vi "signal_mapping_lock-in-measurement.vi"() -> ()   [LabVIEW 2024]
uses:
  <vilib>/Utility/file.llb/Write Delimited Spreadsheet (string).vi
  <vilib>/Utility/file.llb/Write Delimited Spreadsheet (DBL).vi
  <vilib>/Analysis/NI_AALBase.lvlib
panel:
  in  "Set Sensitivities":bool
  in  "A Sensitivity":u16(ring)=20 items=["1 nV/fA", "2 nV/fA", "5 nV/fA", "10 nV/fA", "20 nV/fA", "50 nV/fA", "100 nV/fA", "200 nV/fA", "500 nV/fA", "1 uV/pA", "2 uV/pA", "5 uV/pA", "10 uV/pA", "20 uV/pA", "50 uV/pA", "100 uV/pA", "200 uV/pA", "500 uV/pA", "1 mV/nA", "2 mV/nA", "5 mV/nA", "10 mV/nA", "20 mV/nA", "50 mV/nA", "100 mV/nA", "200 mV/nA", "500 mV/nA", "1 V/uA"]
  in  "B Sensitivity":u16(ring)=20 items=["1 nV/fA", "2 nV/fA", "5 nV/fA", "10 nV/fA", "20 nV/fA", "50 nV/fA", "100 nV/fA", "200 nV/fA", "500 nV/fA", "1 uV/pA", "2 uV/pA", "5 uV/pA", "10 uV/pA", "20 uV/pA", "50 uV/pA", "100 uV/pA", "200 uV/pA", "500 uV/pA", "1 mV/nA", "2 mV/nA", "5 mV/nA", "10 mV/nA", "20 mV/nA", "50 mV/nA", "100 mV/nA", "200 mV/nA", "500 mV/nA", "1 V/uA"]
  in  "Lock-In Num Avgs":i32
  out "错误输出":errorcluster
  out "AUX-ADC4 (V)":sgl format="%.3f"
  out "AUX-ADC3 (V)":sgl format="%.3f"
  out "AUX-ADC1 (V)":sgl format="%.3f"
  out "AUX-ADC2 (V)":sgl format="%.3f"
  in  "OE1022D 2":refnum<visa-resource-name> caption="OE1022D"
  out "序列号":string
  in  "ms to wait after move":u32=1
  in  "ANC300 address":refnum<visa-resource-name>="COM8"
  in  "Snake":bool
  in  "File to save to":path
  in  "Select Scan Type":u16(ring)=1 items=["line scan", "rectangular scan"]
  in  "scan points":i32
  in  "y end":i32
  in  "x end":i32
  in  "y start":i32
  in  "x start":i32
  in  "y scan points":i32
  in  "x scan points":i32
  in  "y scan size":i32
  in  "x scan size":i32
  in  "y center":i32
  in  "x center":i32
  # "Scaning Setup"
  # "Rectangular Scan Parameters"
  # "Line Scan Parameters"
  # "Measurement Setup"
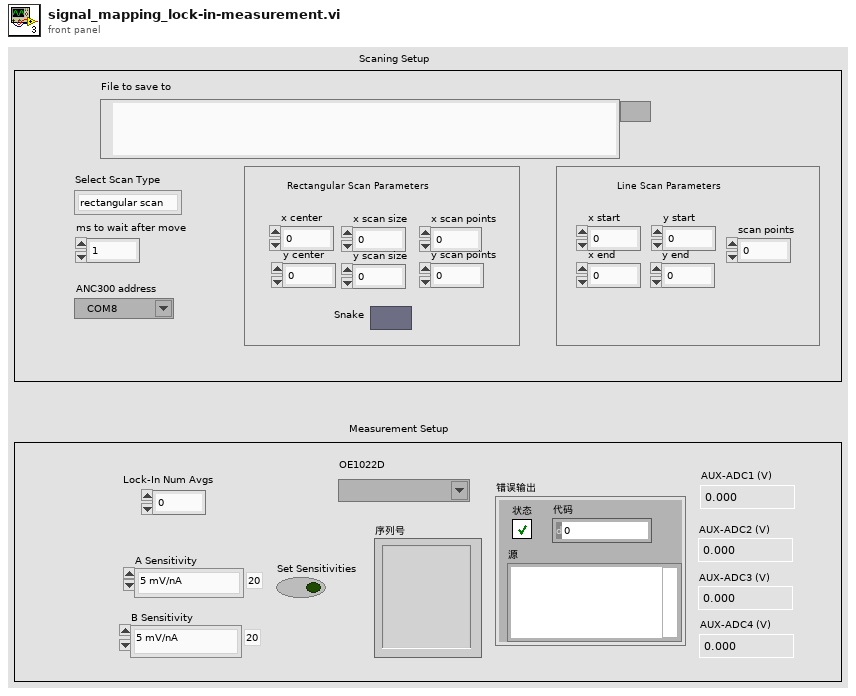
[diagram p1: front panel]
types:
  T1 = cluster{"error ":bool, "error number":i32, "error code":string}
  T2 = cluster{"AD1":dbl[], "AD2":dbl[], "AD3":dbl[], "AD4":dbl[]}
  T3 = cluster{"XB":dbl[], "YB":dbl[], "FrequencyB":dbl[], "NoiseB":dbl[], "Xh1B":dbl[], "Yh1B":dbl[], "Xh2B":dbl[], "Yh2B":dbl[], "Xh2B":dbl[]}
  T4 = cluster{"XA":dbl[], "YA":dbl[], "FrequencyA":dbl[], "NoiseA":dbl[], "Xh1A":dbl[], "Yh1A":dbl[], "Xh2A":dbl[], "Yh2A":dbl[]}
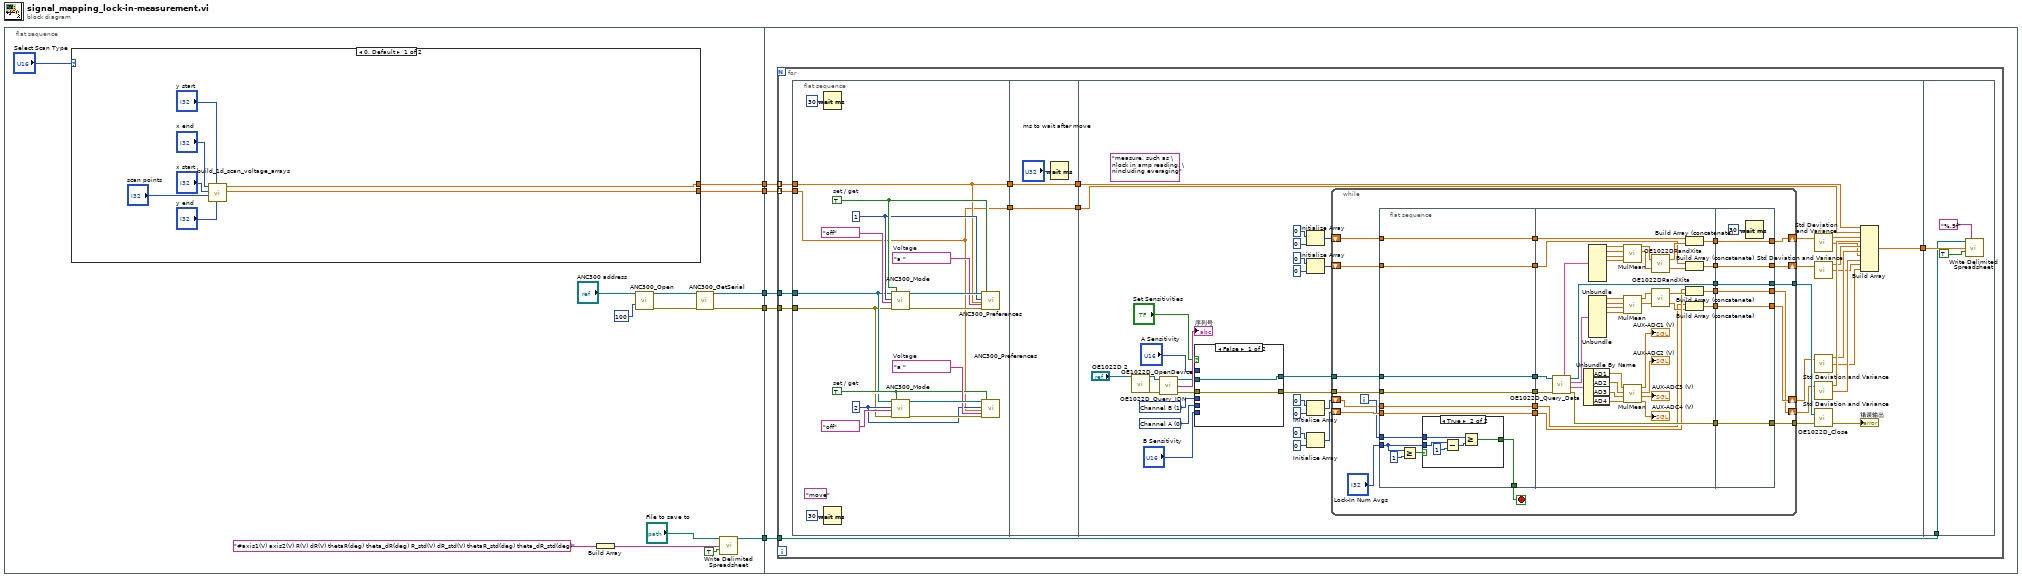
[diagram p0: block diagram]
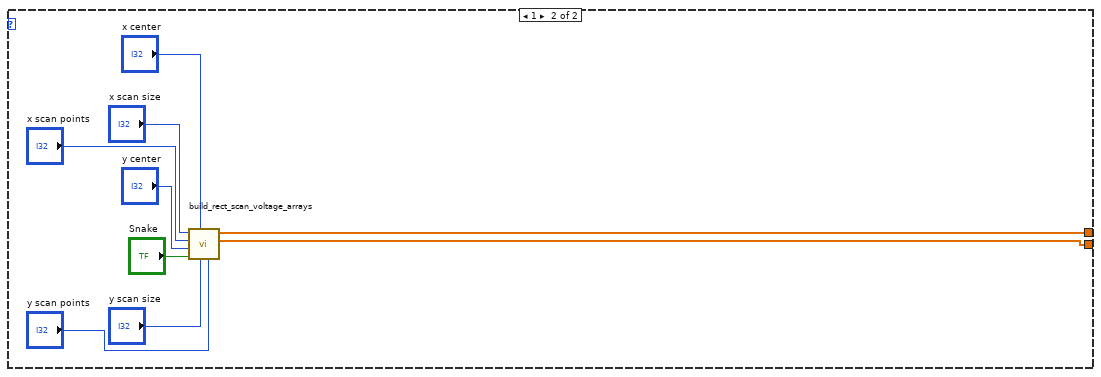
[diagram p2: hidden frame]
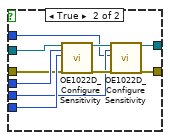
[diagram p3: hidden frame]
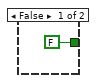
[diagram p4: hidden frame]
diagram:
  n1 = flat-sequence {
    tunnel: [w18] -> w5
    tunnel: [w19] -> w4
    tunnel: [w13] -> w3
    tunnel: [w12] -> w2
    tunnel: [w6] -> w1
    tunnel: w5 -> [w40]
    tunnel: w4 -> [w39]
    tunnel: w3 -> [w38]
    tunnel: w2 -> [w37]
    tunnel: w1 -> [w36]
    frame #0 {
      n2 = case shown="0, Default" "Select Scan Type" {
        tunnel: [w20 w35] -> w19
        tunnel: [w21 w34] -> w18
        frame 0, Default {
          n3 = call "build_1d_scan_voltage_arrays.vi"("y end"="y end", "y start"="y start", "scan points"="scan points", "x start"="x start", "x end"="x end") -> ("y voltage array"=w20:dbl[], "x voltage array"=w21:dbl[])  [unwired: 5 in]
        }
        frame 1 {
          n4 = call "build_rect_scan_voltage_arrays.vi"("y scan points"="y scan points", "y scan size"="y scan size", "x center"="x center", "Snake"="Snake", "y center"="y center", "x scan points"="x scan points", "x scan size"="x scan size") -> ("y voltage array"=w35:dbl[], "x voltage array"=w34:dbl[])  [unwired: 3 in]
        }
      }
      n5 = Build Array("#axis1(V) axis2(V) R(V) dR(V) thetaR(deg) theta_dR(deg) R_std(V) dR_std(V) thetaR_std(deg) theta_dR_std(deg)") -> (w8:string[])
      n6 = call "ANC300_Open.vi"("ANC300 Communication Port In"="ANC300 address", "milliseconds to wait"=u32 100 ("millisecond timer value")) -> ("ANC300 Communication Port Out"=w14:refnum<visa-resource-name>, "error out"=w11:T1)  [unwired: 13 in, 3 out]
      n7 = call "ANC300_GetSerial.vi"("ANC300 Communication Port In"=w14, "error in"=w11) -> ("ANC300 Communication Port Out"=w13:refnum<visa-resource-name>, "error out"=w12:T1)  [unwired: 10 in, 6 out]
      n8 = call-poly <vilib>:"Write Delimited Spreadsheet.vi"("file path (dialog if empty)"="File to save to", "1D data"=w8, "append to file? (new file:F)"=TRUE) -> ("new file path (Not A Path if cancelled)"=w6:path)  [unwired: 11 in, 1 out]
    }
    frame #1 {
      n9 = for {
        tunnel: w40 -> [w50] mode=indexing
        tunnel: w39 -> [w49] mode=indexing
        tunnel: w38 -> [w48]
        tunnel: w37 -> [w47]
        tunnel: w36 -> [w41]
        n10 = flat-sequence {
          tunnel: w50 -> [w52]
          tunnel: w49 -> [w51]
          tunnel: w48 -> [w55]
          tunnel: w47 -> [w54]
          tunnel: [w52] -> w44
          tunnel: [w51] -> w43
          tunnel: [w70] -> w45
          tunnel: w44 -> [w70]
          tunnel: w43 -> [w69]
          tunnel: [w69] -> w42
          tunnel: [w108] -> w46
          tunnel: w45 -> [w100]
          tunnel: w42 -> [w99]
          tunnel: w46 -> [w219]
          tunnel: w41 -> [w217]
          frame #0 {
            w56 = 2
            w57 = 1
            w58 = TRUE  # set / get
            w60 = "a "  # Voltage
            w63 = TRUE  # set / get
            w66 = "a "  # Voltage
            (unwired) "move"
            n11 = Wait (ms)(milliseconds to wait=u32 30 ("2: ms to wait")) -> ()  [unwired: 1 out]
            n12 = Wait (ms)(milliseconds to wait=u32 30 ("1: ms to wait")) -> ()  [unwired: 1 out]
            n13 = call "ANC300_Mode.vi"("ANC300 Communication Port In"=w55, "Axis"=w57, "axis mode in"="off", "error in"=w54, "set / get"=w63) -> ("ANC300 Communication Port Out"=w68:refnum<visa-resource-name>, "error out"=w67:T1)  [unwired: 8 in, 5 out]
            n14 = call "ANC300_Mode.vi"("ANC300 Communication Port In"=w55, "Axis"=w56, "axis mode in"="off", "error in"=w54, "set / get"=w58) -> ("ANC300 Communication Port Out"=w62:refnum<visa-resource-name>, "error out"=w61:T1)  [unwired: 8 in, 5 out]
            n15 = call "ANC300_Preferences.vi"("ANC300 Communication Port In"=w68, "Axis"=w57, "value in"=w52, "parameter"=w66, "error in"=w67, "set / get"=w63) -> ()  [unwired: 6 in, 8 out]
            n16 = call "ANC300_Preferences.vi"("ANC300 Communication Port In"=w62, "Axis"=w56, "value in"=w51, "parameter"=w60, "error in"=w61, "set / get"=w58) -> ()  [unwired: 6 in, 8 out]
          }
          frame #1 {
            n17 = Wait (ms)(milliseconds to wait="ms to wait after move") -> ()  [unwired: 1 out]
          }
          frame #2 {
            w86 = u8 0 items=["Channel A", "Channel B"] ("OE1022D A/B")
            w92 = u8 1 items=["Channel A", "Channel B"] ("OE1022D A/B")
            (unwired) "measure, such as \nlock in amp reading, \nincluding everaging"
            n18 = call "OE1022D_OpenDevice.vi"("VISA resource name"="OE1022D 2") -> ("VISA资源名称输出"=w105:refnum<visa-resource-name>, "错误输出"=w106:errorcluster)  [unwired: 17 in]
            n19 = call "OE1022D_Query_IDN.vi"("错误输入（无错误）"=w106, "VISA resource name"=w105) -> ("错误输出"=w90:errorcluster, "序列号"=→"序列号":string, "VISA resource name out"=w89:refnum<visa-resource-name>)  [unwired: 1 in]
            n20 = case shown="False" "Set Sensitivities" {
              tunnel: w92 -> [_ w126]
              tunnel: "B Sensitivity" -> [_ w125]
              tunnel: w90 -> [w115 w124]
              tunnel: w89 -> [w116 w123]
              tunnel: [w116 w120] -> w88
              tunnel: [w115 w119] -> w87
              tunnel: w86 -> [_ w118]
              tunnel: "A Sensitivity" -> [_ w117]
              frame False {
              }
              frame True {
                n21 = call "OE1022D_Configure Sensitivity.vi"("VISA resource name"=w123, "OE1022D A/B"=w126, "Sensitivity"=w125, "error in (no error)"=w124) -> ("VISA resource name out"=w121:refnum<visa-resource-name>, "error out"=w122:errorcluster)  [unwired: 14 in]
                n22 = call "OE1022D_Configure Sensitivity.vi"("VISA resource name"=w121, "OE1022D A/B"=w118, "Sensitivity"=w117, "error in (no error)"=w122) -> ("VISA resource name out"=w120:refnum<visa-resource-name>, "error out"=w119:errorcluster)  [unwired: 14 in]
              }
            }
            n23 = Initialize Array(0, 0) -> (w114:i32[])
            n24 = Initialize Array(0, 0) -> (w94:i32[])
            n25 = Initialize Array(0, 0) -> (w93:i32[])
            n26 = Initialize Array(0, 0) -> (w109:i32[])
            n27 = while {
              shift-right: [w128] -> w76
              shift-left: w114 -> [w150]
              shift-right: [w129] -> w82
              shift-left: w109 -> [w148]
              tunnel: w87 -> [w140]
              tunnel: w88 -> [w141]
              tunnel: [w139] -> w102
              tunnel: [w138] -> w101
              shift-right: [w134] -> w80
              shift-left: w94 -> [w136]
              shift-right: [w130] -> w78
              shift-left: w93 -> [w133]
              i -> [w143]
              stop <- w142 stop-if-true
              n28 = flat-sequence {
                tunnel: w148 -> [w163]
                tunnel: w150 -> [w164]
                tunnel: [w157] -> w147
                tunnel: [w156] -> w146
                tunnel: [w164] -> w145
                tunnel: [w163] -> w144
                tunnel: w143 -> [w162]
                tunnel: [w161] -> w142
                tunnel: "Lock-In Num Avgs" -> [w159]
                tunnel: w140 -> [w157]
                tunnel: w141 -> [w156]
                tunnel: [w155] -> w137
                tunnel: w136 -> [w155]
                tunnel: w133 -> [w154]
                tunnel: [w154] -> w132
                tunnel: [w207] -> w153
                tunnel: [w206] -> w152
                tunnel: [w183] -> w151
                tunnel: [w180] -> w149
                tunnel: w147 -> [w209]
                tunnel: w146 -> [w208]
                tunnel: w145 -> [w184]
                tunnel: w144 -> [w181]
                tunnel: w137 -> [w176]
                tunnel: [w174] -> w135
                tunnel: w132 -> [w172]
                tunnel: [w171] -> w131
                tunnel: w153 -> [w213]
                tunnel: w152 -> [w212]
                tunnel: [w214] -> w128
                tunnel: w151 -> [w214]
                tunnel: w149 -> [w215]
                tunnel: [w215] -> w129
                tunnel: [w213] -> w139
                tunnel: [w212] -> w138
                tunnel: w135 -> [w211]
                tunnel: [w211] -> w134
                tunnel: w131 -> [w210]
                tunnel: [w210] -> w130
                frame #0 {
                  n29 = Greater Or Equal?(x=w159, y=1) -> (x >= y?=w158:bool)
                  n30 = case shown="True" w158 {
                    tunnel: w162 -> [_ w170]
                    tunnel: [FALSE w169] -> w161
                    tunnel: w159 -> [_ w166]
                    frame False {
                    }
                    frame True {
                      n31 = Subtract(x=w166, y=1) -> (x-y=w167:i32)
                      n32 = Greater Or Equal?(x=w170, y=w167) -> (x >= y?=w169:bool)
                    }
                  }
                }
                frame #1 {
                  n33 = call "OE1022D_Query_Data.vi"("错误输入（无错误）"=w209, "VISA resource name"=w208) -> ("error out"=w207:errorcluster, "输出簇ADC"=w187:T2, "输出簇B"=w186:T3, "VISA resource name out"=w206:refnum<visa-resource-name>, "输出簇A"=w188:T4)  [unwired: 3 in]
                  n34 = Unbundle By Name(w187) -> ("AD1"=w202:dbl[], "AD2"=w203:dbl[], "AD3"=w204:dbl[], "AD4"=w205:dbl[])
                  n35 = Unbundle(w188) -> ("XA"=w193:dbl[], "YA"=w194:dbl[], "FrequencyA"=w195:dbl[], "NoiseA"=w196:dbl[])  [unwired: 4 out]
                  n36 = Unbundle(w186) -> ("XB"=w200:dbl[], "YB"=w199:dbl[], "FrequencyB"=w198:dbl[], "NoiseB"=w197:dbl[])  [unwired: 5 out]
                  n37 = call "MulMean.vi"("IN 4"=w196, "IN 3"=w195, "IN 2"=w194, "IN 1"=w193) -> ("mean 2"=w178:dbl, "mean 1"=w177:dbl)  [unwired: 4 in, 2 out]
                  n38 = call "MulMean.vi"("IN 4"=w197, "IN 3"=w198, "IN 2"=w199, "IN 1"=w200) -> ("mean 2"=w179:dbl, "mean 1"=w201:dbl)  [unwired: 4 in, 2 out]
                  n39 = call "MulMean.vi"("IN 4"=w205, "IN 3"=w204, "IN 2"=w203, "IN 1"=w202) -> ("mean 4"=→"AUX-ADC4 (V)":dbl, "mean 3"=→"AUX-ADC3 (V)":dbl, "mean 2"=→"AUX-ADC2 (V)":dbl, "mean 1"=→"AUX-ADC1 (V)":dbl)  [unwired: 4 in]
                  n40 = call "OE1022DRandXita.vi"("Y"=w178, "X"=w177) -> ("θ (°)"=w175:dbl, "R"=w185:dbl)
                  n41 = call "OE1022DRandXita.vi"("Y"=w179, "X"=w201) -> ("θ (°)"=w173:dbl, "R"=w182:dbl)
                  n42 = Build Array (concatenate)(w184, w185) -> (w183:dbl[])
                  n43 = Build Array (concatenate)(w176, w175) -> (w174:dbl[])
                  n44 = Build Array (concatenate)(w181, w182) -> (w180:dbl[])
                  n45 = Build Array (concatenate)(w172, w173) -> (w171:dbl[])
                }
                frame #2 {
                  n46 = Wait (ms)(milliseconds to wait=30) -> ()  [unwired: 1 out]
                }
              }
            }
            n47 = call <vilib>:"Std Deviation and Variance.vi"("X"=w76) -> ("mean"=w83:dbl, "standard deviation"=w75:dbl)  [unwired: 1 in, 1 out]
            n48 = call <vilib>:"Std Deviation and Variance.vi"("X"=w80) -> ("mean"=w79:dbl, "standard deviation"=w73:dbl)  [unwired: 1 in, 1 out]
            n49 = call <vilib>:"Std Deviation and Variance.vi"("X"=w78) -> ("mean"=w77:dbl, "standard deviation"=w72:dbl)  [unwired: 1 in, 1 out]
            n50 = call <vilib>:"Std Deviation and Variance.vi"("X"=w82) -> ("mean"=w81:dbl, "standard deviation"=w74:dbl)  [unwired: 1 in, 1 out]
            n51 = call "OE1022D_Close.vi"("错误输入（无错误）"=w102, "VISA resource name"=w101) -> ("错误输出"=→"错误输出":errorcluster)  [unwired: 1 in]
            n52 = Build Array(w100, w99, w83, w81, w79, w77, w75, w74, w73, w72) -> (w108:dbl[])
          }
          frame #3 {
            n53 = call-poly <vilib>:"Write Delimited Spreadsheet.vi"("file path (dialog if empty)"=w217, "format (%.3f)"="%.9f", "1D data"=w219, "append to file? (new file:F)"=TRUE) -> ()  [unwired: 10 in, 2 out]
          }
        }
      }
    }
  }
